vi "Main Title.vi"(8 "Error In":errorcluster) -> (0 "Error Out":errorcluster)   [LabVIEW 2019, in "Controller.lvlib"]
uses:
  Controller.lvlib
  Queues/Queues.lvlib
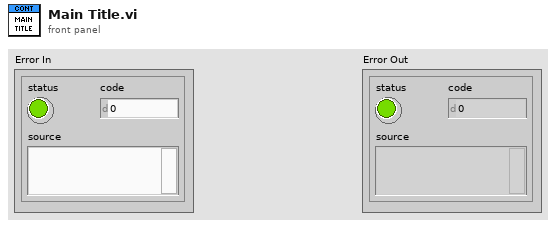
[diagram p1: front panel]
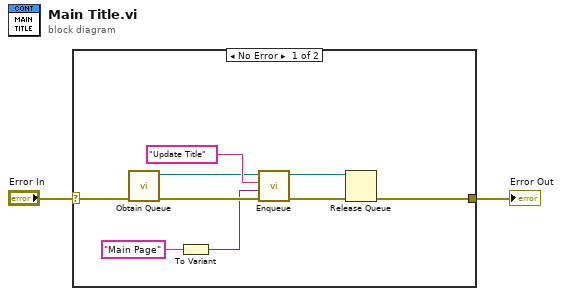
[diagram p0: block diagram]
diagram:
  n1 = case shown="No Error" "Error In" {
    selector: "Error In" -> [w10 w12]
    tunnel: [w5 w12] -> w2
    frame No Error {
      n2 = call "Obtain Queue.vi"("Error In"=w10) -> ("Error Out"=w9:errorcluster, "Queue out"=w8:refnum<queue>)  [unwired: 9 in]
      n3 = To Variant(anything="Main Page") -> (Variant=w4:variant)
      n4 = call "Enqueue.vi"("Error In"=w9, "Data"=w4, "State"="Update Title", "Queue in"=w8) -> ("Error Out"=w7:errorcluster, "Queue out"=w6:refnum<queue>)  [unwired: 6 in]
      n5 = Release Queue(queue=w6, error in (no error)=w7) -> (error out=w5:errorcluster)  [unwired: 1 in, 2 out]
    }
    frame Error {
    }
  }
  "Error Out" <- w2
